vi "ParsesCANFDFrame.vi"(10 "CANFD数据帧数组":T1(array[cluster])) -> (1 "CANFD报文显示":string[][](table), 3 "CANFD数据帧数组(out)":T1(array[cluster]))   [LabVIEW 2013]
panel:
  in  "空数组输入":u8[](array[numeric])
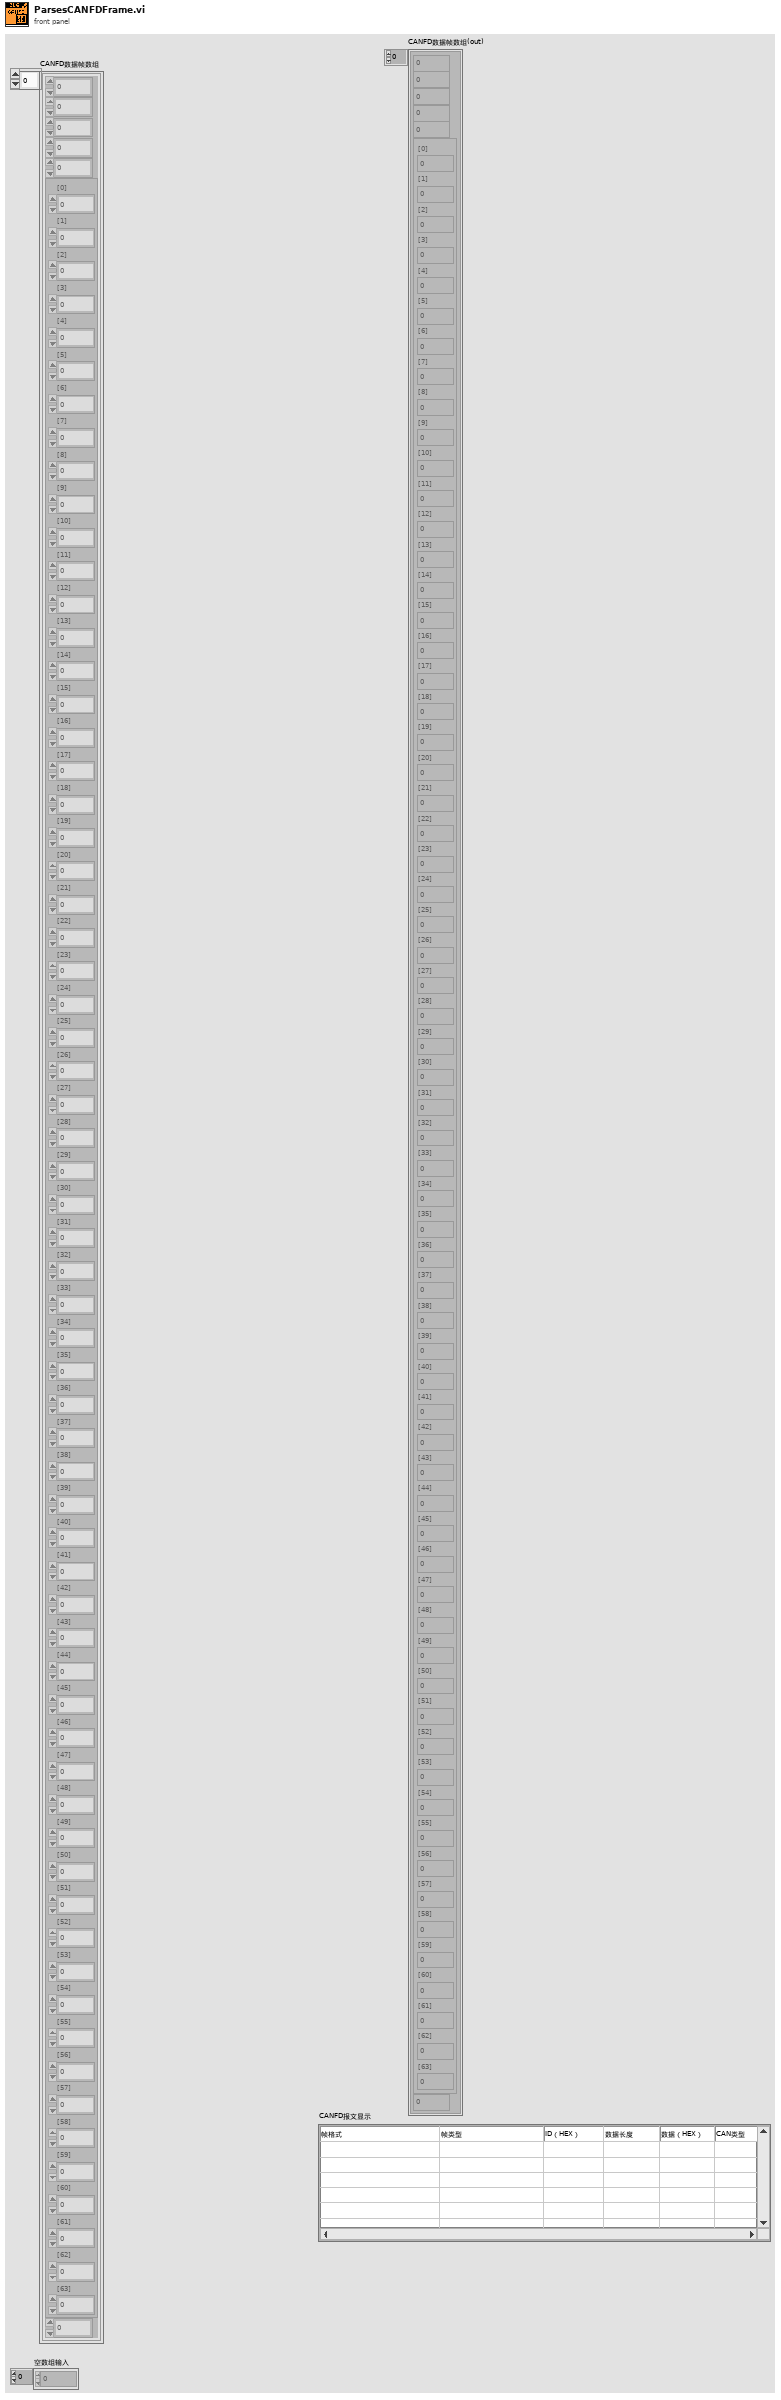
[diagram p1: front panel]
types:
  T1 = cluster{u32, u8, u8, u8, u8, cluster{"[0]":u8, "[1]":u8, "[2]":u8, "[3]":u8, "[4]":u8, "[5]":u8, "[6]":u8, "[7]":u8, "[8]":u8, "[9]":u8, "[10]":u8, "[11]":u8, "[12]":u8, "[13]":u8, "[14]":u8, "[15]":u8, "[16]":u8, "[17]":u8, "[18]":u8, "[19]":u8, "[20]":u8, "[21]":u8, "[22]":u8, "[23]":u8, "[24]":u8, "[25]":u8, "[26]":u8, "[27]":u8, "[28]":u8, "[29]":u8, "[30]":u8, "[31]":u8, "[32]":u8, "[33]":u8, "[34]":u8, "[35]":u8, "[36]":u8, "[37]":u8, "[38]":u8, "[39]":u8, "[40]":u8, "[41]":u8, "[42]":u8, "[43]":u8, "[44]":u8, "[45]":u8, "[46]":u8, "[47]":u8, "[48]":u8, "[49]":u8, "[50]":u8, "[51]":u8, "[52]":u8, "[53]":u8, "[54]":u8, "[55]":u8, "[56]":u8, "[57]":u8, "[58]":u8, "[59]":u8, "[60]":u8, "[61]":u8, "[62]":u8, "[63]":u8}, u64}[]
  T2 = cluster{"[0]":u8, "[1]":u8, "[2]":u8, "[3]":u8, "[4]":u8, "[5]":u8, "[6]":u8, "[7]":u8, "[8]":u8, "[9]":u8, "[10]":u8, "[11]":u8, "[12]":u8, "[13]":u8, "[14]":u8, "[15]":u8, "[16]":u8, "[17]":u8, "[18]":u8, "[19]":u8, "[20]":u8, "[21]":u8, "[22]":u8, "[23]":u8, "[24]":u8, "[25]":u8, "[26]":u8, "[27]":u8, "[28]":u8, "[29]":u8, "[30]":u8, "[31]":u8, "[32]":u8, "[33]":u8, "[34]":u8, "[35]":u8, "[36]":u8, "[37]":u8, "[38]":u8, "[39]":u8, "[40]":u8, "[41]":u8, "[42]":u8, "[43]":u8, "[44]":u8, "[45]":u8, "[46]":u8, "[47]":u8, "[48]":u8, "[49]":u8, "[50]":u8, "[51]":u8, "[52]":u8, "[53]":u8, "[54]":u8, "[55]":u8, "[56]":u8, "[57]":u8, "[58]":u8, "[59]":u8, "[60]":u8, "[61]":u8, "[62]":u8, "[63]":u8}
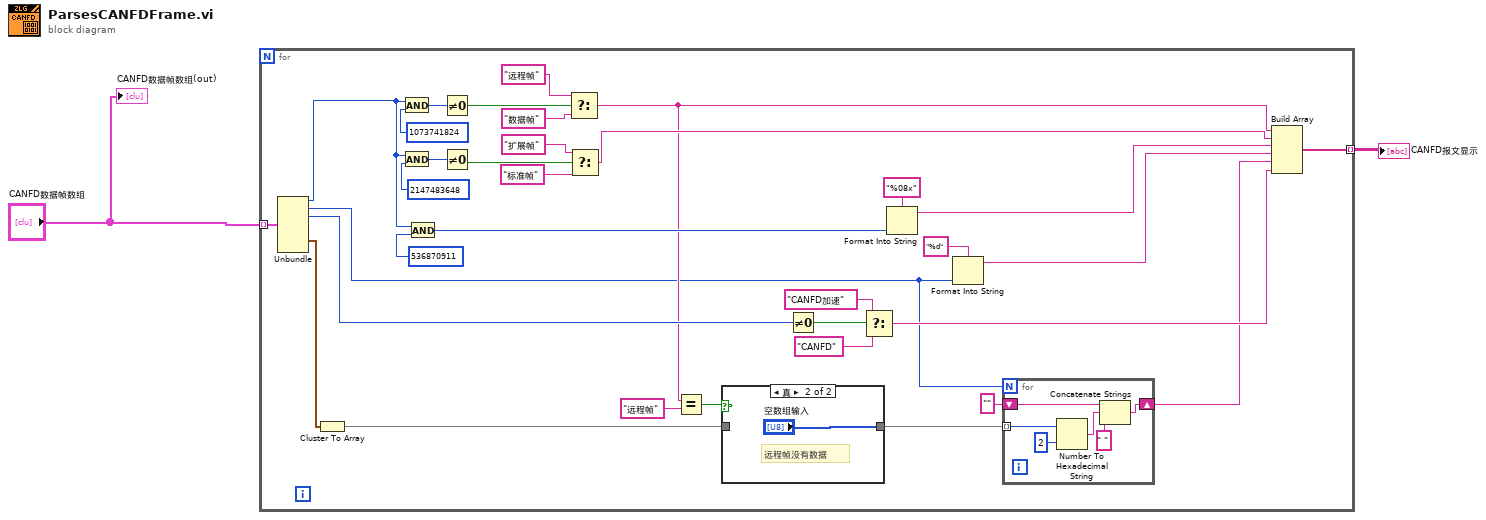
[diagram p0: block diagram]
diagram:
  n1 = for {
    tunnel: "CANFD数据帧数组" -> [w20] mode=indexing
    tunnel: [w13] -> w1 mode=indexing
    n2 = Unbundle(w20) -> (w31:u32, w5:u8, w12:u8, w30:T2)  [unwired: 3 out]
    n3 = Cluster To Array(cluster=w30) -> (array=w21:u8[])
    n4 = And(x=w31, y=u32 1073741824) -> (x .and. y?=w32:u32)
    n5 = And(x=w31, y=u32 2147483648) -> (x .and. y?=w33:u32)
    n6 = And(x=w31, y=u32 536870911) -> (x .and. y?=w17:u32)
    n7 = Not Equal To 0?(x=w32) -> (x != 0?=w25:bool)
    n8 = Not Equal To 0?(x=w33) -> (x != 0?=w24:bool)
    n9 = Select(t="远程帧", s=w25, f="数据帧") -> (s? t:f=w7:string)
    n10 = Select(t="扩展帧", s=w24, f="标准帧") -> (s? t:f=w16:string)
    n11 = Equal?(x=w7, y="远程帧") -> (x = y?=w22:bool)
    n12 = case shown="真" w22 {
      tunnel: [w43 "空数组输入"] -> w4
      tunnel: w21 -> [w43 _]
      frame False {
      }
      frame True {
        # "远程帧没有数据"
      }
    }
    n13 = Not Equal To 0?(x=w12) -> (x != 0?=w11:bool)
    n14 = Select(t="CANFD加速", s=w11, f="CANFD") -> (s? t:f=w8:string)
    n15 = Format Into String(format string="%08x", w17) -> (resulting string=w15:string)  [unwired: 2 in, 1 out]
    n16 = Format Into String(format string="%d", w5) -> (resulting string=w14:string)  [unwired: 2 in, 1 out]
    n17 = for {
      N: w5 -> [_]
      shift-right: [w39] -> w3
      shift-left: "" -> [w37]
      tunnel: w4 -> [w38] mode=indexing
      n18 = Number To Hexadecimal String(1:i16 2 ("width (-)"), 2:w38) -> (0:w41:string)
      n19 = Concatenate Strings(w37, w41, " " ("string")) -> (w39:string)
    }
    n20 = Build Array(w7, w16, w15, w14, w3, w8) -> (w13:string[])
  }
  "CANFD报文显示" <- w1
  "CANFD数据帧数组(out)" <- "CANFD数据帧数组"
